vi "CSC_SetGravityDirection.vi"(4 "Trans_Gto0":T1=[[1.0, 0.0, 0.0, 0.0], [0.0, 1.0, 0.0, 0.0], [0.0, 0.0, 1.0, 0.0], [0.0, 0.0, 0.0, 1.0]], 6 "Gravity Direction (empty)\n!!Function Not Tested!!":dbl[](array[numeric]), 8 "error in (no error)":errorcluster, 9 "Negative Direction (T)":bool=TRUE, 10 "Gravity Axis in G (Z)":T2=enum."Z", 11 "CSC in":refnum<class "CableSerialChain.lvclass">) -> (0 "error out":errorcluster, 3 "CSC out":refnum<class "CableSerialChain.lvclass">)   [LabVIEW 2015, in "CableSerialChain.lvclass"]
uses:
  CableSerialChain.lvclass
  Body/xyzO.ctl
  <vilib>/Analysis/Matrix/Datatypes/RealMatrix.ctl
  <vilib>/Analysis/baseanly.llb/Matrix Type of Inverse Matrix.ctl
  CableSerialChain.lvclass/CableSerialChain.ctl
  <vilib>/Analysis/baseanly.llb/Real Inverse Matrix.vi
  <vilib>/Analysis/BLAS.llb/dgemv - General Matrix-Vector Product (DBL).vi
  <vilib>/Analysis/NI_AALBLAS.lvlib
  <vilib>/Analysis/NI_AALBase.lvlib
  Body/Bodies.lvclass
  <vilib>/Analysis/Matrix/NI_Matrix.lvlib
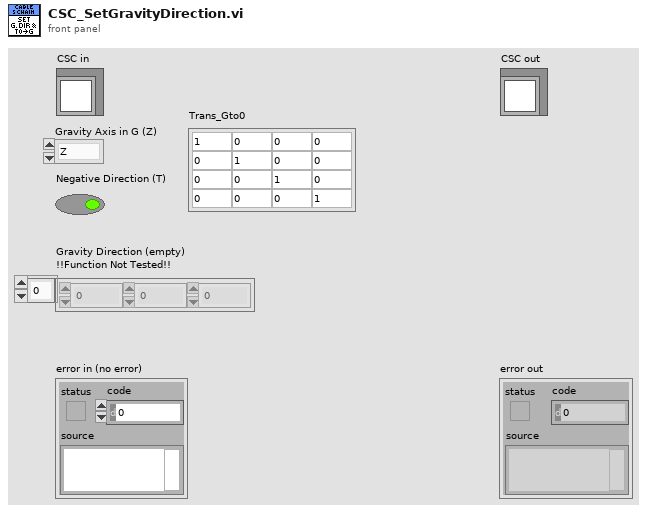
[diagram p1: front panel]
types:
  T1 = typedef "NI_Matrix.lvlib/RealMatrix.ctl" = dbl[][]
  T2 = typedef "Bodies.lvclass/xyzO.ctl" = enum16{"X", "Y", "Z", "O"}
  T3 = typedef "NI_AALBase.lvlib/Matrix Type of Inverse Matrix.ctl" = enum32{"General", "Positive Definite", "Lower Triangular", "Upper Triangular"}
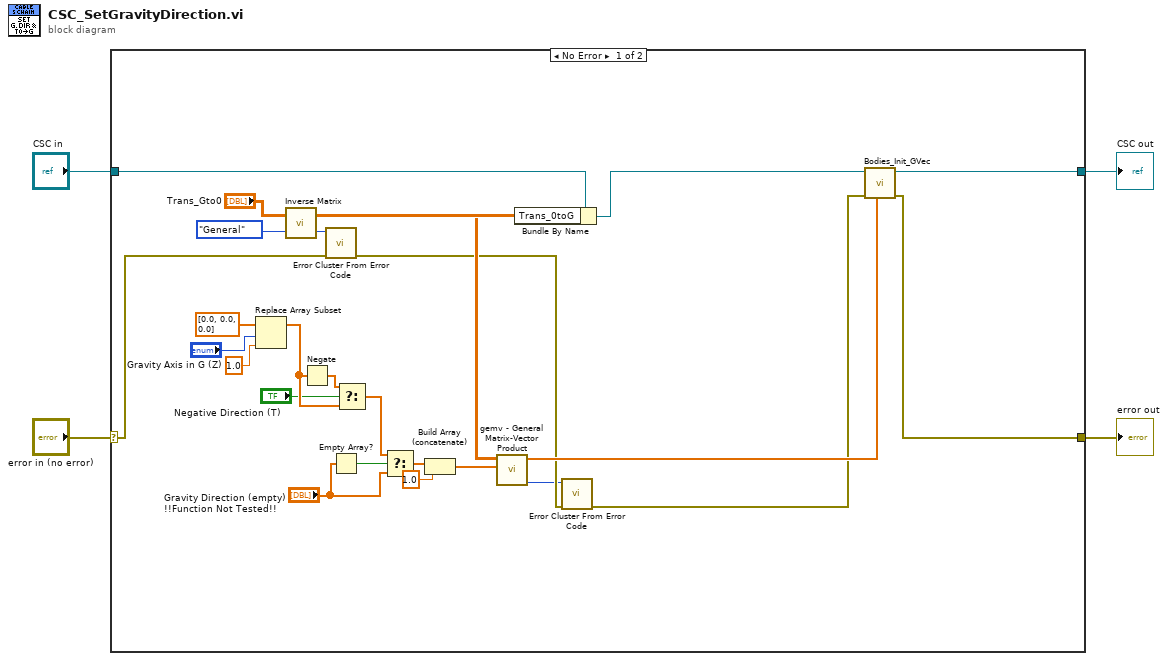
[diagram p0: block diagram]
diagram:
  n1 = case shown="No Error" "error in (no error)" {
    selector: "error in (no error)" -> [w28 w31]
    tunnel: [w24 w31] -> w3
    tunnel: [w5 w30] -> w1
    tunnel: "CSC in" -> [w29 w30]
    frame No Error {
      n2 = Replace Array Subset(array=dbl[] [0.0, 0.0, 0.0], new element=1.0 ("new element/subarray"), index="Gravity Axis in G (Z)") -> (w18:dbl[])
      n3 = call-poly <vilib>:"Inverse Matrix.vi"("matrix type"=Matrix_Type_of_Inverse_Matrix."General", "Input Matrix"="Trans_Gto0") -> ("error"=w20:i32, "Inverse Matrix"=w22:T1)
      n4 = Negate(x=w18) -> (-x=w17:dbl[])
      n5 = call <vilib>:"Error Cluster From Error Code.vi"("error in (no error)"=w28, "error code (0)"=w20) -> ("error out"=w19:errorcluster)  [unwired: 7 in]
      n6 = Empty Array?(array="Gravity Direction (empty)\n!!Function Not Tested!!") -> (empty?=w9:bool)
      n7 = Select(t=w17, s="Negative Direction (T)", f=w18) -> (s? t:f=w8:dbl[])
      n8 = Select(t=w8, s=w9, f="Gravity Direction (empty)\n!!Function Not Tested!!") -> (s? t:f=w6:dbl[])
      n9 = Build Array (concatenate)(w6, 1.0) -> (w10:dbl[])
      n10 = call-poly <vilib>:"gemv - General Matrix-Vector Product.vi"("x"=w10, "A"=w22) -> ("error"=w12:i32, "dgemv"=w26:dbl[])  [unwired: 8 in]
      n11 = Bundle By Name(cluster=w29, "Trans_0toG"="Trans_Gto0") -> (w27:refnum<class "CableSerialChain.lvclass">)
      n12 = call <vilib>:"Error Cluster From Error Code.vi"("error in (no error)"=w19, "error code (0)"=w12) -> ("error out"=w25:errorcluster)  [unwired: 7 in]
      n13 = call-dynamic "Bodies_Init_GVec.vi"("Gravity Direction"=w26, "error in (no error)"=w25, "Bodies in"=w27) -> ("error out"=w24:errorcluster, "Bodies out"=w5:refnum<class "CableSerialChain.lvclass">)  [unwired: 7 in]
    }
    frame Error {
    }
  }
  "error out" <- w3
  "CSC out" <- w1
